vi "Close.vi"(8 "error in (no error)":errorcluster, 11 "DLL in":refnum<class "NI_AB_API_PPL.lvclass">) -> (0 "error out":errorcluster)   [LabVIEW 2020, in "NI_AB_API_PPL.lvclass"]
uses:
  <vilib>/AppBuilder/AB_API/PPL/NI_AB_API_PPL.lvclass
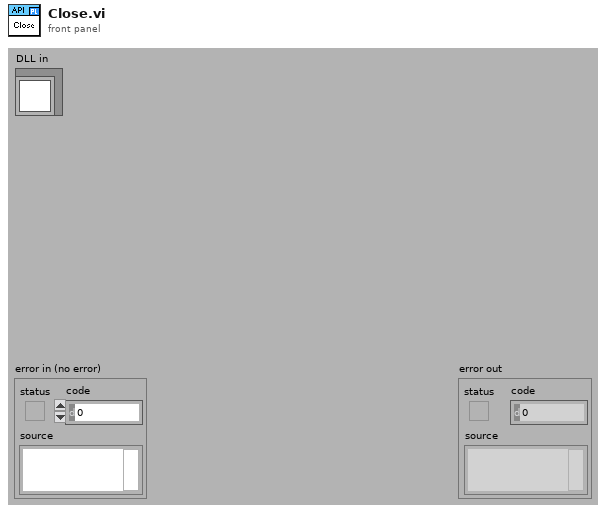
[diagram p1: front panel]
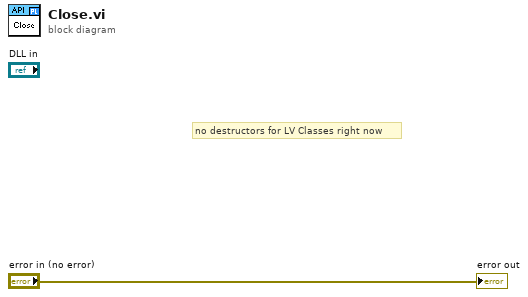
[diagram p0: block diagram]
diagram:
  # "no destructors for LV Classes right now"
  "error out" <- "error in (no error)"
